vi "global_config.vi"() -> ()   [LabVIEW 2015]
panel:
  out "默认上传数据输出":string[](array[string])
  out "配置信息输出":T1
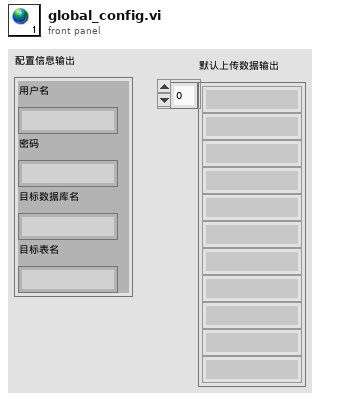
[diagram p1: front panel]
types:
  T1 = cluster{"用户名":string, "密码":string, "目标数据库名":string, "目标表名":string}
diagram:
